vi "Save DAC Configuration.vi"(8 "error in":errorcluster, 10 "Config File refnum in":T1, 11 "DAC in":refnum<class "DAC.lvclass">) -> (0 "error out":errorcluster, 2 "Config File refnum out":T1, 3 "DAC out":refnum<class "DAC.lvclass">)   [LabVIEW 2019, in "DAC.lvlib" / "DAC.lvclass"]
uses:
  DAC.lvclass
  <vilib>/Utility/config.llb/Config Data RefNum.ctl
  DAC.lvclass/DAC.ctl
  <vilib>/Utility/config.llb/Write Key (Boolean).vi
  <vilib>/Utility/config.llb/Write Key (String).vi
  <vilib>/Utility/config.llb/Write Key (Double).vi
  <vilib>/Utility/config.llb/NI_LVConfig.lvlib
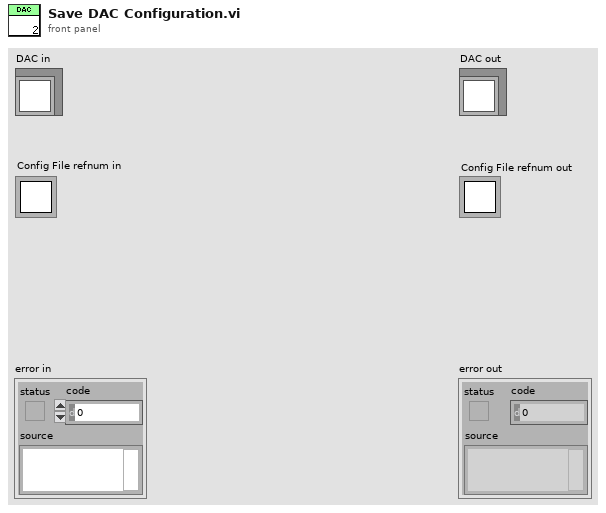
[diagram p1: front panel]
types:
  T1 = typedef "NI_LVConfig.lvlib/Config Data RefNum.ctl" = refnum<k1>
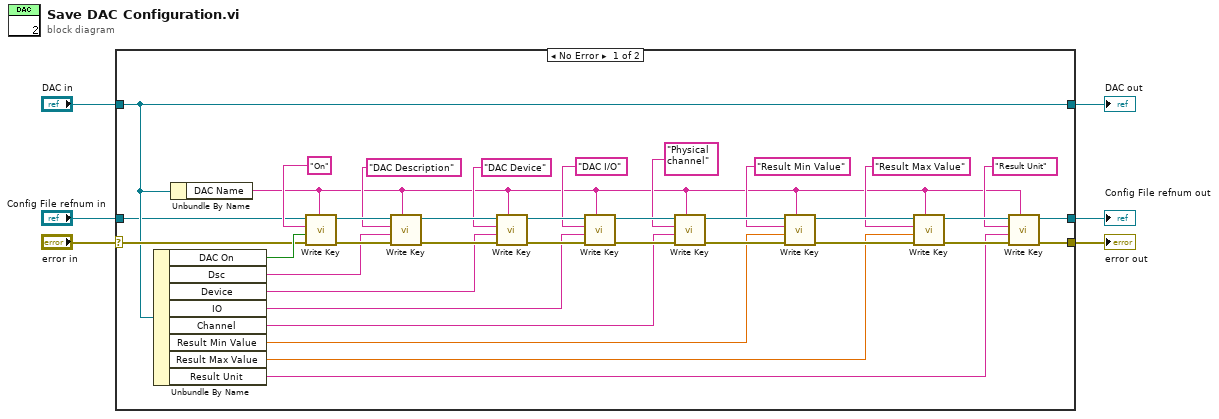
[diagram p0: block diagram]
diagram:
  n1 = case shown="No Error" "error in" {
    selector: "error in" -> [w40 w45]
    tunnel: [w20 w45] -> w5
    tunnel: [w39 w44] -> w3
    tunnel: "DAC in" -> [w39 w44]
    tunnel: "Config File refnum in" -> [w38 w43]
    tunnel: [w27 w43] -> w1
    frame No Error {
      n2 = Unbundle By Name(w39) -> ("DAC On"=w41:bool, "Dsc"=w34:string, "Device"=w12:string, "IO"=w11:string, "Channel"=w10:string, "Result Min Value"=w9:dbl, "Result Max Value"=w8:dbl, "Result Unit"=w7:string)
      n3 = Unbundle By Name(w39) -> ("DAC Name"=w13:string)
      n4 = call-poly <vilib>:"Write Key.vi"("section"=w13, "error in (no error)"=w40, "value"=w41, "key"="On", "refnum"=w38) -> ("error out"=w36:errorcluster, "refnum out"=w37:T1)  [unwired: 4 in, 1 out]
      n5 = call-poly <vilib>:"Write Key.vi"("section"=w13, "error in (no error)"=w36, "value"=w34, "key"="DAC Description", "refnum"=w37) -> ("error out"=w26:errorcluster, "refnum out"=w33:T1)  [unwired: 4 in, 1 out]
      n6 = call-poly <vilib>:"Write Key.vi"("section"=w13, "error in (no error)"=w26, "value"=w12, "key"="DAC Device", "refnum"=w33) -> ("error out"=w25:errorcluster, "refnum out"=w32:T1)  [unwired: 4 in, 1 out]
      n7 = call-poly <vilib>:"Write Key.vi"("section"=w13, "error in (no error)"=w25, "value"=w11, "key"="DAC I/O", "refnum"=w32) -> ("error out"=w24:errorcluster, "refnum out"=w31:T1)  [unwired: 4 in, 1 out]
      n8 = call-poly <vilib>:"Write Key.vi"("section"=w13, "error in (no error)"=w24, "value"=w10, "key"="Physical channel", "refnum"=w31) -> ("error out"=w23:errorcluster, "refnum out"=w30:T1)  [unwired: 4 in, 1 out]
      n9 = call-poly <vilib>:"Write Key.vi"("section"=w13, "error in (no error)"=w23, "value"=w9, "key"="Result Min Value", "refnum"=w30) -> ("error out"=w22:errorcluster, "refnum out"=w29:T1)  [unwired: 4 in, 1 out]
      n10 = call-poly <vilib>:"Write Key.vi"("section"=w13, "error in (no error)"=w22, "value"=w8, "key"="Result Max Value", "refnum"=w29) -> ("error out"=w21:errorcluster, "refnum out"=w28:T1)  [unwired: 4 in, 1 out]
      n11 = call-poly <vilib>:"Write Key.vi"("section"=w13, "error in (no error)"=w21, "value"=w7, "key"="Result Unit", "refnum"=w28) -> ("error out"=w20:errorcluster, "refnum out"=w27:T1)  [unwired: 4 in, 1 out]
    }
    frame Error {
    }
  }
  "error out" <- w5
  "DAC out" <- w3
  "Config File refnum out" <- w1
